vi "Measure.vi"(0 "Instrument handle":refnum<k15>[](array[refnum]), 1 "Measurements":T2[](array[typedef]), 2 "Compliance Check Duration":dbl=0.0001 format="%#_13g", 5 "Channel Name":string[](array[string]), 7 "Compliance Skip Duration":dbl[](array[numeric]) format="%.6p", 9 "Aperture Time":dbl[](array[numeric]) format="%#_13g", 11 "error in (no error)":errorcluster, 12 "Pin Name":string[](array[string]), 13 "Log Configurations":T1) -> (4 "Measurements":T2[](array[typedef]), 6 "Measure complete?":bool[](array[boolean]), 8 "Error List[]":string[](array[string]), 15 "error out":errorcluster)   [LabVIEW 2024, in "devicePowerSequencerCoreLogic.lvlib"]
uses:
  devicePowerSequencerCoreLogic.lvlib
  controls/Voltage and Current Measurements.ctl
  controls/Log Configurations.ctl
  Form Error Message.vi/4da3fa3f-d6a2-4c6b-9c9c-fc44bca91f7b.vi
  <vilib>/Utility/error.llb/Error Cluster From Error Code.vi
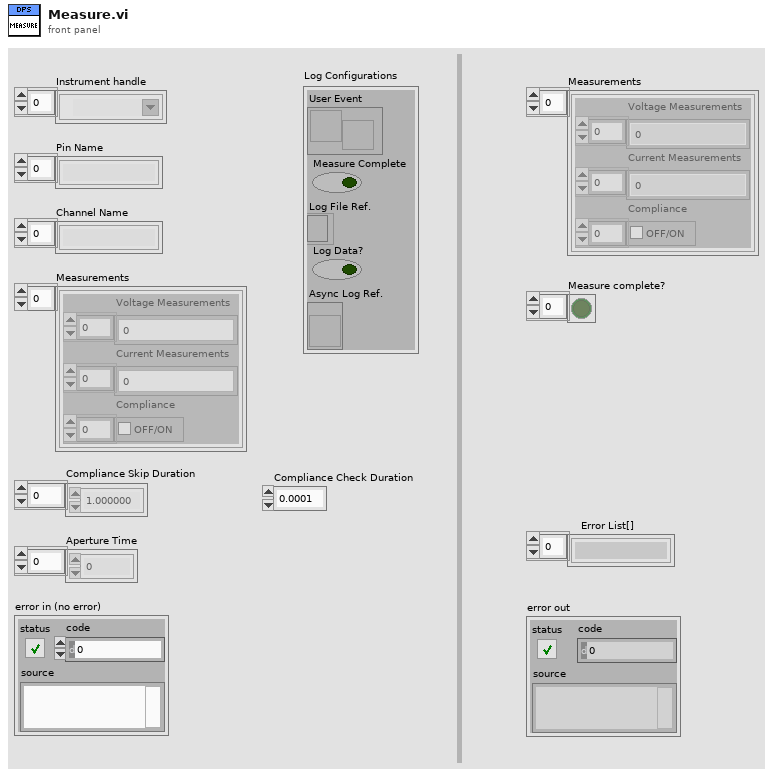
[diagram p1: front panel]
types:
  T1 = typedef "devicePowerSequencerCoreLogic.lvlib/Log Configurations.ctl" = cluster{"User Event":refnum<user-event>, "Measure Complete":bool, "Log File Ref.":refnum<file>, "Log Data?":bool, "Async Log Ref.":refnum<vi>}
  T2 = typedef "devicePowerSequencerCoreLogic.lvlib/Voltage and Current Measurements.ctl" = cluster{"Voltage Measurements":dbl[], "Current Measurements":dbl[], "Compliance":bool[]}
  T3 = cluster{"Measured Data":cluster{"Voltage":dbl[], "Current":dbl[]}[], "Measure Complete":bool}
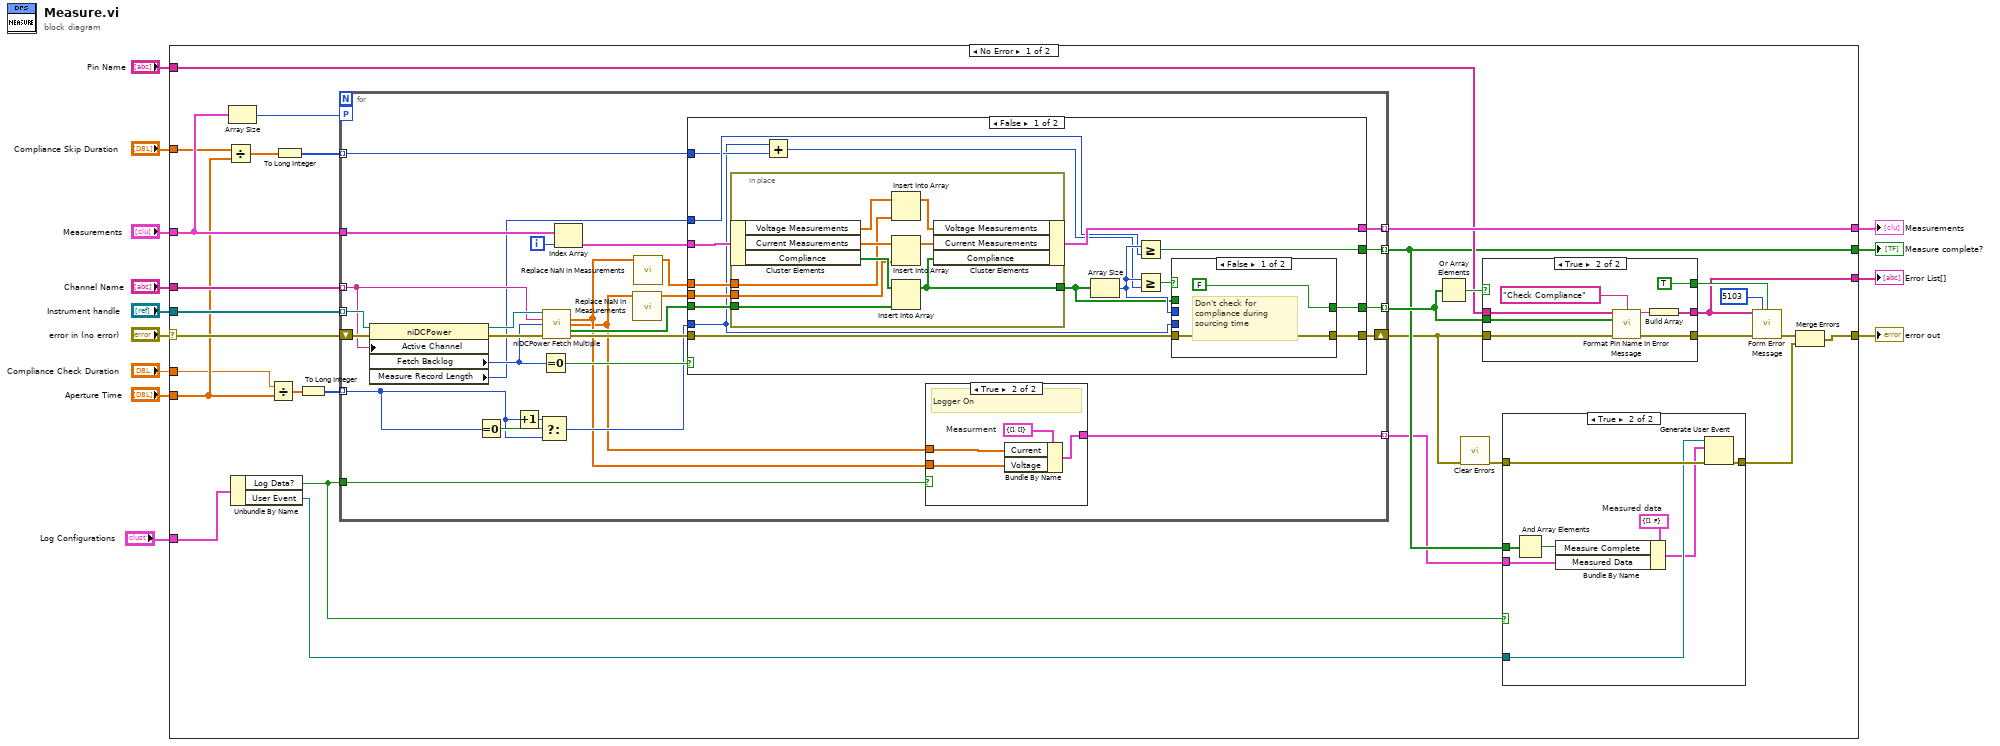
[diagram p0: block diagram]
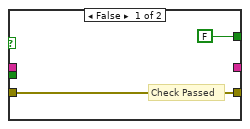
[diagram p2: hidden frame]
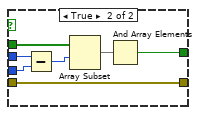
[diagram p4: hidden frame]
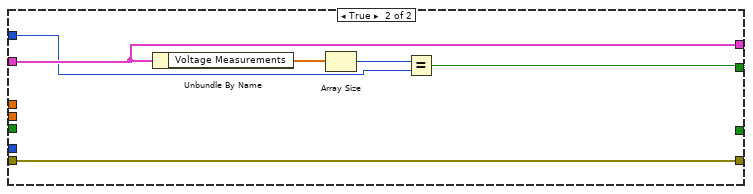
[diagram p5: hidden frame]
diagram:
  n1 = case shown="No Error" "error in (no error)" {
    selector: "error in (no error)" -> [w37 w135]
    tunnel: "Measurements" -> [w43 _]
    tunnel: "Channel Name" -> [w41 _]
    tunnel: "Instrument handle" -> [w40 _]
    tunnel: "Pin Name" -> [w26 _]
    tunnel: [w19 w135] -> w9
    tunnel: [w24 _] -> w8
    tunnel: [w38 _] -> w7
    tunnel: "Aperture Time" -> [w32 _]
    tunnel: "Compliance Skip Duration" -> [w33 _]
    tunnel: [w21 _] -> w3
    tunnel: "Log Configurations" -> [w22 _]
    tunnel: "Compliance Check Duration" -> [w14 _]
    frame No Error {
      n2 = Divide(x=w33, y=w32) -> (x/y=w34:dbl[])
      n3 = Array Size(array=w43) -> (size(s)=w42:i32)
      n4 = Unbundle By Name(w22) -> ("Log Data?"=w15:bool, "User Event"=w16:refnum<user-event>)
      n5 = Divide(x=w14, y=w32) -> (x/y=w36:dbl[])
      n6 = To Long Integer(number=w34) -> (32bit integer=w31:i32[])
      n7 = To Long Integer(number=w36) -> (32bit integer=w35:i32[])
      n8 = for {
        tunnel: w40 -> [w80] mode=indexing
        tunnel: w41 -> [w72] mode=indexing
        shift-right: [w78] -> w20
        shift-left: w37 -> [w81]
        tunnel: [w79] -> w24 mode=indexing
        tunnel: w43 -> [w77]
        workers-P: w42 -> [_]
        tunnel: [w69] -> w38 mode=indexing
        tunnel: w35 -> [w59] mode=indexing
        tunnel: w31 -> [w65] mode=indexing
        tunnel: [w64] -> w28 mode=indexing
        tunnel: [w63] -> w23 mode=indexing
        tunnel: w15 -> [w62]
        i -> [w76]
        n9 = property class="niDCPower"(reference=w80, error in=w81, "Active Channel"=w72) -> (reference out=w74:refnum<k15>, error out=w73:errorcluster, "Fetch Backlog"=w71:i32, "Measure Record Length"=w67:i32)
        n10 = Equal To 0?(x=w59) -> (x = 0?=w61:bool)
        n11 = Increment(x=w59) -> (x+1=w58:i32)
        n12 = Select(t=w58, s=w61, f=w59) -> (s? t:f=w60:i32)
        n13 = Equal To 0?(x=w71) -> (x = 0?=w66:bool)
        n14 = call <instrlib>:"niDCPower Fetch Multiple.vi"("instrument handle"=w74, "channel name"=w72, "count (1)"=w71, "error in (no error)"=w73) -> ("voltage measurements"=w55:dbl[], "current measurements"=w54:dbl[], "in compliance"=w68:bool[], "error out"=w70:errorcluster)  [unwired: 6 in, 2 out]
        n15 = Index Array(array=w77, index=w76) -> (element=w75:T2)
        n16 = call "Replace NaN in Measurements.vi"("Measurements"=w54) -> ("Measurements"=w56:dbl[])  [unwired: 14 in]
        n17 = call "Replace NaN in Measurements.vi"("Measurements"=w55) -> ("Measurements"=w57:dbl[])  [unwired: 14 in]
        n18 = case shown="False" w66 {
          tunnel: [w101 w120] -> w79
          tunnel: [w98 w125] -> w78
          tunnel: w75 -> [w97 w124]
          tunnel: w70 -> [w95 w125]
          tunnel: [w94 w124] -> w69
          tunnel: w68 -> [w93 _]
          tunnel: w56 -> [w92 _]
          tunnel: w57 -> [w91 _]
          tunnel: w60 -> [w86 _]
          tunnel: w67 -> [w90 w121]
          tunnel: w65 -> [w88 _]
          tunnel: [w87 _] -> w64
          frame False {
            n19 = in-place {
              in-place-border: [w107] -> w96
              in-place-border: w93 -> [w104]
              in-place-border: w92 -> [w102]
              in-place-border: w91 -> [w103]
              n20 = in-place-cluster #1(w97) -> ("Voltage Measurements"=w110:dbl[], "Current Measurements"=w105:dbl[], "Compliance"=w106:bool[])
              n21 = Insert Into Array(array=w110, new element=w103) -> (w109:dbl[])  [unwired: 1 in]
              n22 = Insert Into Array(array=w105, new element=w102) -> (w108:dbl[])  [unwired: 1 in]
              n23 = Insert Into Array(array=w106, new element=w104) -> (w107:bool[])  [unwired: 1 in]
              n24 = in-place-cluster #1("Voltage Measurements"=w109, "Current Measurements"=w108, "Compliance"=w107) -> (w94:T2)
            }
            n25 = Add(x=w86, y=w88) -> (x+y=w89:i32)
            n26 = Array Size(array=w96) -> (size(s)=w100:i32)
            n27 = Greater Or Equal?(x=w100, y=w90) -> (x >= y?=w101:bool)
            n28 = Greater Or Equal?(x=w100, y=w89) -> (x >= y?=w99:bool)
            n29 = case shown="False" w99 {
              tunnel: w96 -> [_ w118]
              tunnel: w100 -> [_ w116]
              tunnel: w86 -> [_ w115]
              tunnel: w95 -> [w112 w114]
              tunnel: [w112 w114] -> w98
              tunnel: [FALSE w113] -> w87
              frame False {
                # "Don't check for compliance during sourcing time"
              }
              frame True {
                n30 = Subtract(x=w116, y=w115) -> (x-y=w119:i32)
                n31 = Array Subset(array=w118, index=w119) -> (w117:bool[])  [unwired: 1 in]
                n32 = And Array Elements(Boolean array=w117) -> (logical AND=w113:bool)
              }
            }
          }
          frame True {
            n33 = Unbundle By Name(w124) -> ("Voltage Measurements"=w123:dbl[])
            n34 = Array Size(array=w123) -> (size(s)=w122:i32)
            n35 = Equal?(x=w122, y=w121) -> (x = y?=w120:bool)
          }
        }
        n36 = case shown="True" w62 {
          tunnel: [_ w84] -> w63
          tunnel: w54 -> [_ w83]
          tunnel: w55 -> [_ w82]
          frame False {
            # "Logger Off"
          }
          frame True {
            w85 = cluster{"Voltage":dbl[], "Current":dbl[]} {"Voltage"=[], "Current"=[]}  # Measurment
            # "Logger On"
            n37 = Bundle By Name(cluster=w85, "Current"=w83, "Voltage"=w82) -> (w84:cluster{"Voltage":dbl[], "Current":dbl[]})
          }
        }
      }
      n38 = Or Array Elements(Boolean array=w28) -> (logical OR=w27:bool)
      n39 = call <vilib>:"Clear Errors.vi"("error in (no error)"=w20) -> ("error out"=w17:errorcluster)  [unwired: 5 in, 1 out]
      n40 = case shown="True" w27 {
        tunnel: w20 -> [w45 w53]
        tunnel: [w45 w51] -> w29
        tunnel: [_ w50] -> w21
        tunnel: w28 -> [_ w49]
        tunnel: [FALSE ("Boolean") TRUE ("Boolean")] -> w30
        tunnel: w26 -> [_ w46]
        frame False {
          # "Check Passed"
        }
        frame True {
          n41 = call "Format Pin Name In Error Message.vi"("Pin Name"=w46, "Parameter Name"="Check Compliance", "Error[]"=w49, "error in"=w53) -> ("Error Message"=w52:string, "error out"=w51:errorcluster)  [unwired: 10 in]
          n42 = Build Array(w52) -> (w50:string[])
        }
      }
      n43 = case shown="True" w15 {
        tunnel: [w126 w133] -> w25
        tunnel: w17 -> [w126 w134]
        tunnel: w16 -> [_ w132]
        tunnel: w24 -> [_ w128]
        tunnel: w23 -> [_ w131]
        frame False {
        }
        frame True {
          w130 = T3 {"Measured Data"=[], "Measure Complete"=FALSE}  # Measured data
          n44 = And Array Elements(Boolean array=w128) -> (logical AND=w127:bool)
          n45 = Bundle By Name(cluster=w130, "Measure Complete"=w127, "Measured Data"=w131) -> (w129:T3)
          n46 = Generate User Event(user event=w132, event data cluster=w129, error in=w134) -> (error out=w133:errorcluster)  [unwired: 1 in, 1 out]
        }
      }
      n47 = call "Form Error Message.vi"("Error Message"=w21, "error code (0)"=5103, "Error?"=w30, "error in (no error)"=w29) -> ("error out"=w18:errorcluster)  [unwired: 11 in]
      n48 = Merge Errors(w18, w25) -> (w19:errorcluster)
    }
    frame Error {
    }
  }
  "error out" <- w9
  "Measure complete?" <- w8
  "Measurements" <- w7
  "Error List[]" <- w3
